vi "SwerveConfig_Set.vi"   [LabVIEW 2018]
types:
  T1 = enum16{"open", "replace", "create", "open or create", "replace or create", "replace or create with confirmation"}
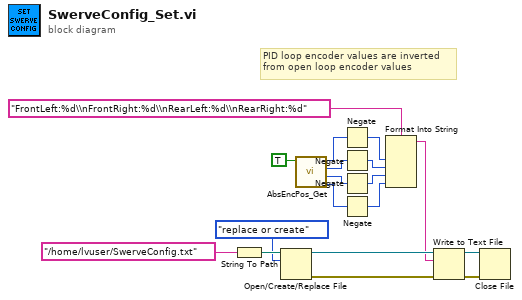
[diagram p0: block diagram]
diagram:
  # "PID loop encoder values are inverted from open loop encoder values"
  n1 = String To Path(string="/home/lvuser/SwerveConfig.txt" ("directory path")) -> (path=w16:path)
  n2 = Open/Create/Replace File(file path (use dialog)=w16, operation (0:open)=T1."replace or create") -> (refnum out=w14:refnum<file>, error out=w13:errorcluster)  [unwired: 4 in, 1 out]
  n3 = call "AbsEncPos_Get.vi"("Update?"=TRUE) -> ("RearRightPulsePos"=w8:i32, "RearLeftPulsePos"=w6:i32, "FrontRightPulsePos"=w7:i32, "FrontLeftPulsePos"=w9:i32)  [unwired: 7 in]
  n4 = Negate(x=w9) -> (-x=w3:i32)
  n5 = Negate(x=w7) -> (-x=w4:i32)
  n6 = Negate(x=w6) -> (-x=w5:i32)
  n7 = Negate(x=w8) -> (-x=w2:i32)
  n8 = Format Into String(format string="FrontLeft:%d\\nFrontRight:%d\\nRearLeft:%d\\nRearRight:%d", w3, w4, w5, w2) -> (resulting string=w11:string)  [unwired: 2 in, 1 out]
  n9 = Write to Text File(file (use dialog)=w14, text=w11, error in=w13) -> (refnum out=w17:refnum<file>, error out=w12:errorcluster)  [unwired: 1 in, 1 out]
  n10 = Close File(refnum=w17, error in=w12) -> ()  [unwired: 2 out]
